vi "error_handler.vi"(8 "error in (no error)":errorcluster, 10 "body":string, 11 "headers":string) -> (0 "error out":errorcluster)   [LabVIEW 2015, in "lv-dropbox.lvlib"]
uses:
  lv-dropbox.lvlib
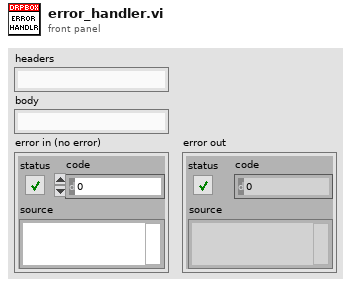
[diagram p1: front panel]
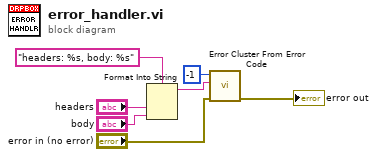
[diagram p0: block diagram]
diagram:
  n1 = Format Into String(format string="headers: %s, body: %s", "headers", "body") -> (resulting string=w4:string)  [unwired: 2 in, 1 out]
  n2 = call <vilib>:"Error Cluster From Error Code.vi"("error in (no error)"="error in (no error)", "error message (\"\")"=w4, "error code (0)"=-1) -> ("error out"=→"error out":errorcluster)  [unwired: 6 in]
